vi "RTS Door Schedule Location.vi"(5 "Station":u8=1 min=1 max=8 step=1, 7 "File Name":string, 8 "error in (no error)":errorcluster, 10 "Input":T1, 11 "Stripped Path Input":path) -> (0 "error out":errorcluster, 2 "Output":T1, 3 "Stripped Path Output":path)   [LabVIEW 2020]
uses:
  Type Definitions/RTS Test Pattern.ctl
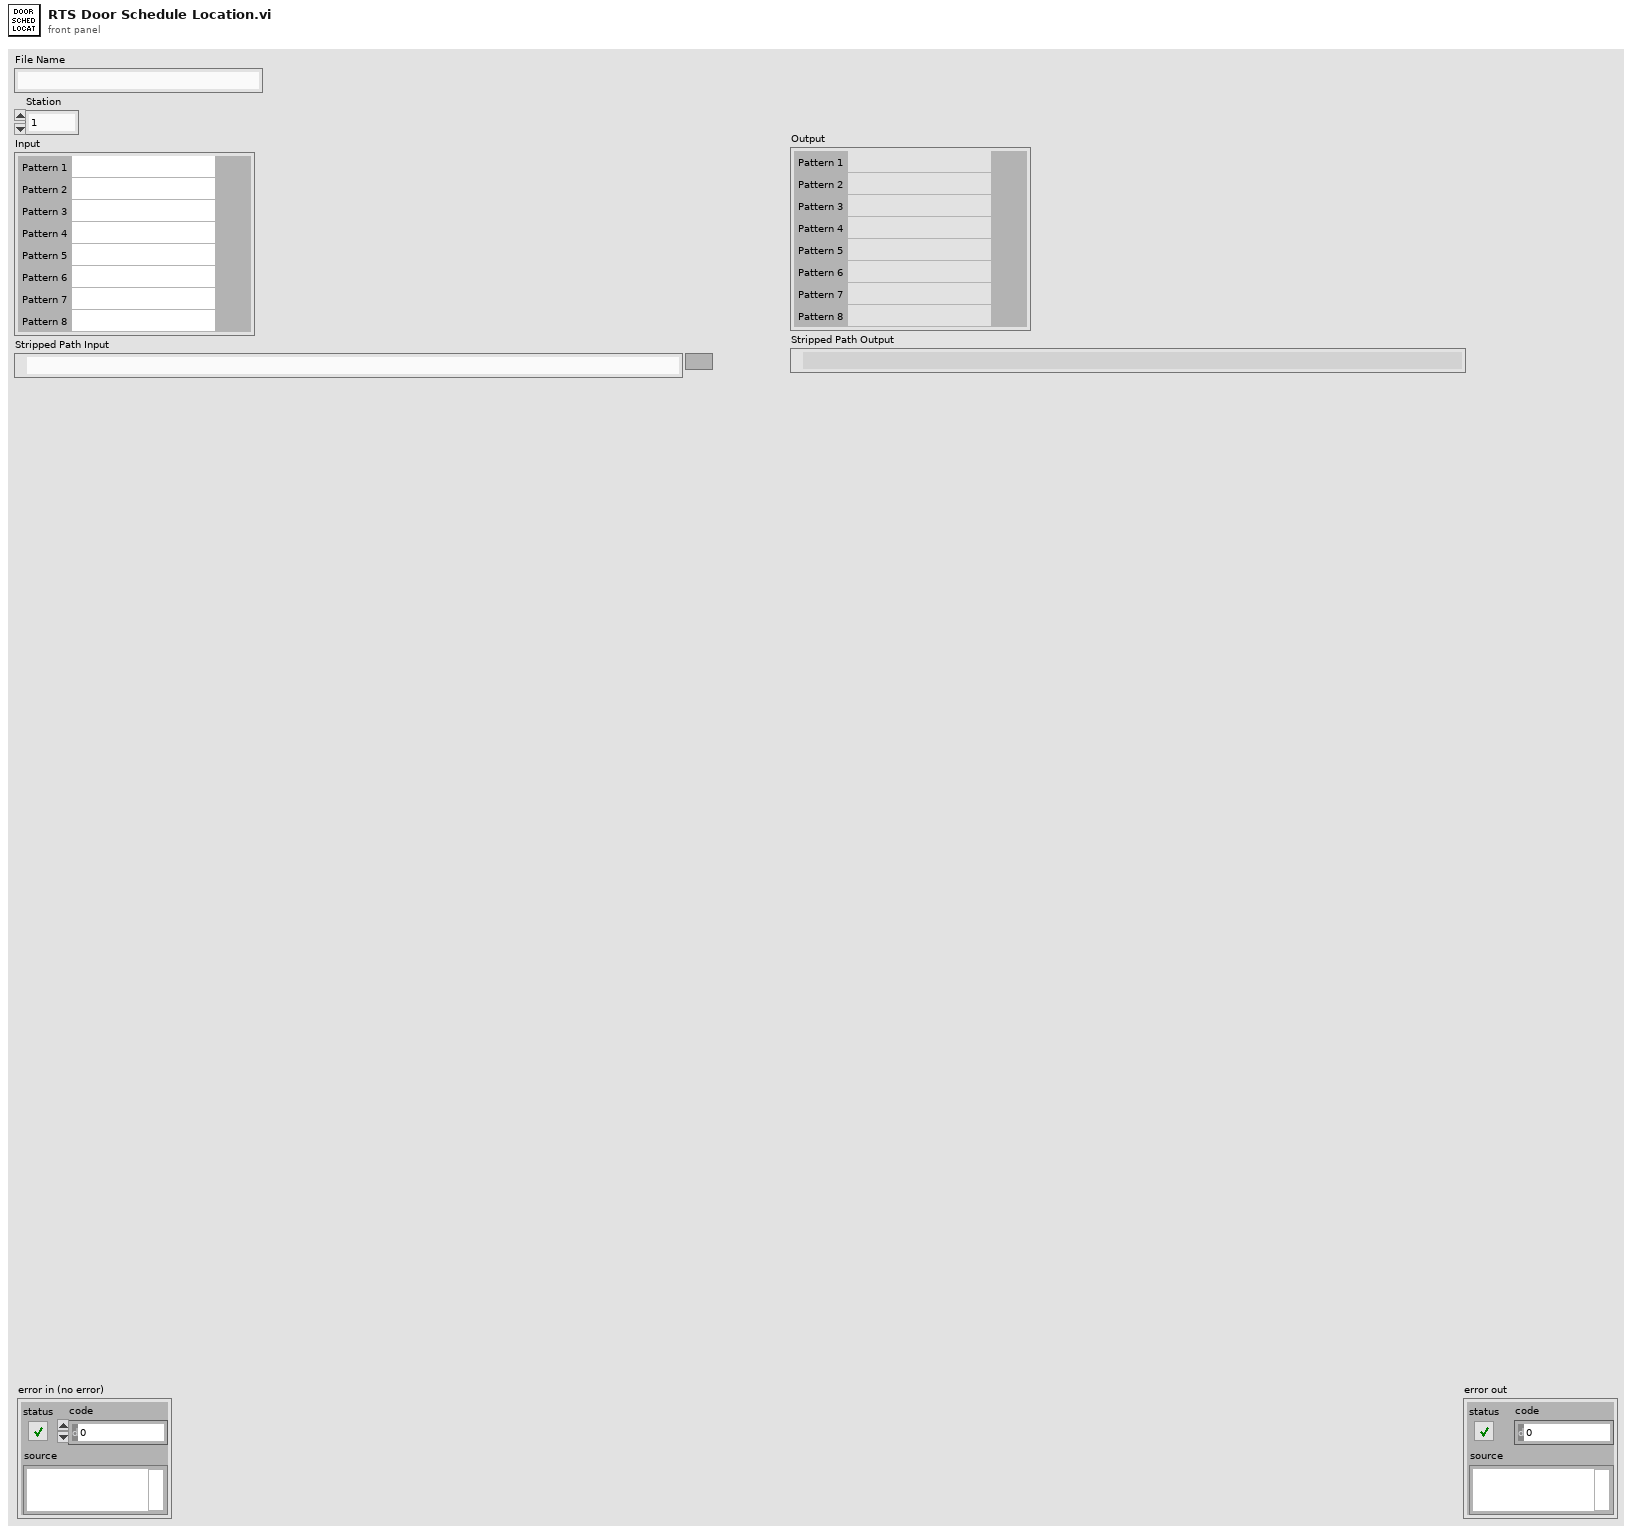
[diagram p1: front panel]
types:
  T1 = typedef "RTS Test Pattern.ctl" = cluster{" Pattern 1":path, "Pattern 2":path, "Pattern 3":path, "Pattern 4":path, "Pattern 5":path, "Pattern 6":path, "Pattern 7":path, "Pattern 8":path}
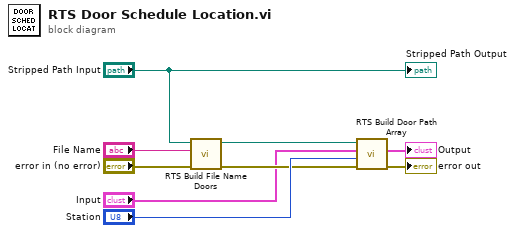
[diagram p0: block diagram]
diagram:
  n1 = call "RTS Build File Name Doors.vi"("error in (no error)"="error in (no error)", "File Name"="File Name", "Stripped Path Input"="Stripped Path Input") -> ("error out"=w6:errorcluster, "appended path"=w4:path)  [unwired: 7 in]
  n2 = call "RTS Build Door Path Array.vi"("Error In"=w6, "Station"="Station", "Input"="Input", "Full Door Ops Path"=w4) -> ("Error Out"=→"error out":errorcluster, "Output"=→"Output":T1)  [unwired: 6 in]
  "Stripped Path Output" <- "Stripped Path Input"
